vi "多列表转换.vi"(10 "多列列表框":refnum<vi>) -> (2 "输出数组":T1(array[cluster]), 3 "是否剩余":bool)   [LabVIEW 2016]
panel:
  out "值":i32
  out "数组":u8[](array[numeric])
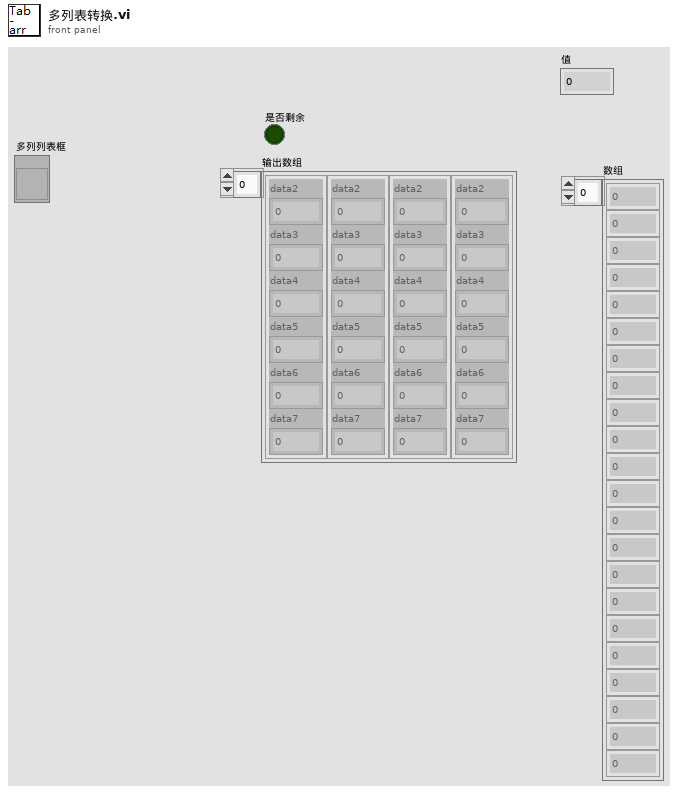
[diagram p1: front panel]
types:
  T1 = cluster{"data2":u8, "data3":u8, "data4":u8, "data5":u8, "data6":u8, "data7":u8}[]
  T2 = cluster{"data2":u8, "data3":u8, "data4":u8, "data5":u8, "data6":u8, "data7":u8}
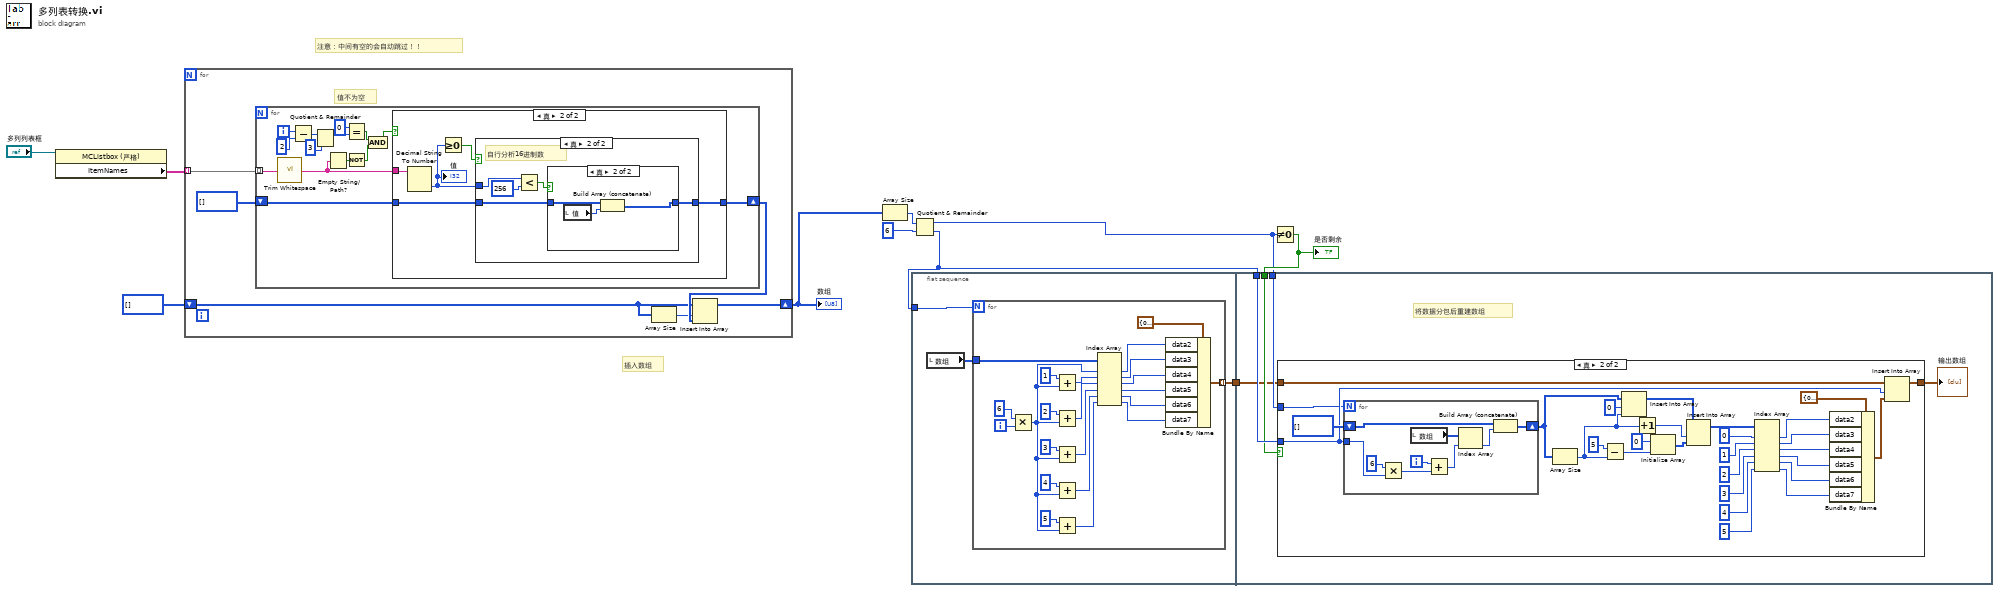
[diagram p0: block diagram]
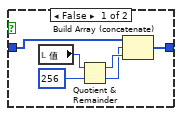
[diagram p5: hidden frame]
diagram:
  # "注意：中间有空的会自动跳过！！"
  # "插入数组"
  n1 = property class="MCListbox (严格)"(reference="多列列表框") -> ("ItemNames"=w1:string[][])  [unwired: 1 in, 2 out]
  n2 = for {
    tunnel: w1 -> [w16] mode=indexing
    shift-right: [w11] -> w7
    shift-left: i32[] [] -> [w13]
    # "值不为空"
    n3 = for {
      tunnel: w16 -> [w23] mode=indexing
      shift-right: [w22] -> w14
      shift-left: i32[] [] -> [w24]
      i -> [w30]
      n4 = call <vilib>:"Trim Whitespace.vi"("string"=w23) -> ("trimmed string"=w21:string)  [unwired: 1 in]
      n5 = Subtract(x=w30, y=2) -> (x-y=w28:i32)
      n6 = Quotient & Remainder(x=w28, y=3) -> (x-y*floor(x/y)=w26:i32)  [unwired: 1 out]
      n7 = Empty String/Path?(string/path=w21) -> (empty?=w20:bool)
      n8 = Equal?(x=0, y=w26) -> (x = y?=w18:bool)
      n9 = Not(x=w20) -> (.not. x?=w19:bool)
      n10 = And(x=w18, y=w19) -> (x .and. y?=w17:bool)
      n11 = case shown="真" w17 {
        tunnel: w21 -> [_ w36]
        tunnel: w24 -> [w31 w33]
        tunnel: [w31 w32] -> w22
        frame False {
        }
        frame True {
          n12 = Decimal String To Number(string=w36) -> (number=w34:i32)  [unwired: 2 in, 1 out]
          "值" <- w34
          n13 = Greater Or Equal To 0?(x=w34) -> (x >= 0?=w35:bool)
          n14 = case shown="真" w35 {
            tunnel: w34 -> [_ w42]
            tunnel: [w37 w39] -> w32
            tunnel: w33 -> [w37 w38]
            frame False {
            }
            frame True {
              # "自行分析16进制数"
              n15 = Less?(x=w42, y=256) -> (x < y?=w40:bool)
              n16 = case shown="真" w40 {
                tunnel: [w48 w49] -> w39
                tunnel: w38 -> [w47 w51]
                frame False {
                  n17 = local read "值"() -> (w46:i32)
                  n18 = Quotient & Remainder(x=w46, y=256) -> (x-y*floor(x/y)=w44:i32, floor(x/y)=w43:i32)
                  n19 = Build Array (concatenate)(w47, w43, w44) -> (w48:i32[])
                }
                frame True {
                  n20 = local read "值"() -> (w50:i32)
                  n21 = Build Array (concatenate)(w51, w50) -> (w49:i32[])
                }
              }
            }
          }
        }
      }
    }
    n22 = Array Size(array=w13) -> (size(s)=w12:i32)
    n23 = Insert Into Array(array=w13, index=w12, new element=w14) -> (w11:i32[])
  }
  "数组" <- w7
  n24 = Array Size(array=w7) -> (size(s)=w9:i32)
  n25 = flat-sequence {
    tunnel: w5 -> [w52]
    tunnel: [w53] -> w6
    tunnel: w6 -> [w78]
    tunnel: w5 -> [w81]
    tunnel: w4 -> [w80]
    tunnel: w3 -> [w79]
    frame #0 {
      n26 = local read "数组"() -> (w54:u8[])
      n27 = for {
        N: w52 -> [_]
        tunnel: w54 -> [w75]
        tunnel: [w55] -> w53 mode=indexing
        i -> [w68]
        n28 = Multiply(x=6, y=w68) -> (x*y=w56:i32)
        n29 = Add(x=1, y=w56) -> (x+y=w57:i32)
        n30 = Add(x=2, y=w56) -> (x+y=w64:i32)
        n31 = Add(x=3, y=w56) -> (x+y=w63:i32)
        n32 = Add(x=4, y=w56) -> (x+y=w61:i32)
        n33 = Add(x=5, y=w56) -> (x+y=w59:i32)
        n34 = Index Array(array=w75, index #1=w56, index #2=w57, index #3=w64, index #4=w63, index #5=w61, index #6=w59) -> (element #1=w74:u8, element #2=w73:u8, element #3=w72:u8, element #4=w71:u8, element #5=w70:u8, element #6=w69:u8)
        n35 = Bundle By Name(cluster=T2 {"data2"=0, "data3"=0, "data4"=0, "data5"=0, "data6"=0, "data7"=0} ("簇"), "data2"=w74, "data3"=w73, "data4"=w72, "data5"=w71, "data6"=w70, "data7"=w69) -> (w55:T2)
      }
    }
    frame #1 {
      # "将数据分包后重建数组"
      n36 = case shown="真" w80 {
        tunnel: w81 -> [_ w90]
        tunnel: [w82 w91] -> w77
        tunnel: w79 -> [_ w89]
        tunnel: w78 -> [w82 w88]
        frame False {
        }
        frame True {
          n37 = for {
            N: w89 -> [_]
            tunnel: w90 -> [w117]
            shift-right: [w115] -> w87
            shift-left: u8[] [] -> [w114]
            i -> [w116]
            n38 = Multiply(x=6, y=w117) -> (x*y=w119:i32)
            n39 = local read "数组"() -> (w113:u8[])
            n40 = Add(x=w116, y=w119) -> (x+y=w118:i32)
            n41 = Index Array(array=w113, index=w118) -> (element=w112:u8)
            n42 = Build Array (concatenate)(w114, w112) -> (w115:u8[])
          }
          n43 = Array Size(array=w87) -> (size(s)=w83:i32)
          n44 = Subtract(x=5, y=w83) -> (x-y=w108:i32)
          n45 = Insert Into Array(array=w87, index=0 ("索引"), new element=w83) -> (w85:u8[])
          n46 = Increment(x=w83) -> (x+1=w84:i32)
          n47 = Initialize Array(0, w108) -> (w107:i32[])
          n48 = Insert Into Array(array=w85, index=w84, new element=w107) -> (w105:u8[])
          n49 = Index Array(array=w105, index #1=0 ("索引"), index #2=1 ("索引"), index #3=2 ("索引"), index #4=3 ("索引"), index #5=4 ("索引"), index #6=5 ("索引")) -> (element #1=w98:u8, element #2=w97:u8, element #3=w96:u8, element #4=w95:u8, element #5=w94:u8, element #6=w93:u8)
          n50 = Bundle By Name(cluster=T2 {"data2"=0, "data3"=0, "data4"=0, "data5"=0, "data6"=0, "data7"=0} ("簇"), "data2"=w98, "data3"=w97, "data4"=w96, "data5"=w95, "data6"=w94, "data7"=w93) -> (w92:T2)
          n51 = Insert Into Array(array=w88, index=w90, new element=w92) -> (w91:T1)
        }
      }
      "输出数组" <- w77
    }
  }
  n52 = Quotient & Remainder(x=w9, y=6) -> (x-y*floor(x/y)=w3:i32, floor(x/y)=w5:i32)
  n53 = Not Equal To 0?(x=w3) -> (x != 0?=w4:bool)
  "是否剩余" <- w4
